vi "Initialize Acquisition.vi"(8 "error in":errorcluster, 11 "DAQmxChannel":T1) -> (0 "error out":errorcluster, 3 "task out":refnum<k21>)   [LabVIEW 2018]
doc: "Konfiguruje kana³ pomiarowy karty DAQ do pomiaru napiêcia."
uses:
  controls/daqtypedef.ctl
  <vilib>/DAQmx/create/channels.llb/DAQmx Create Channel (AI-Voltage-Basic).vi
  <vilib>/DAQmx/configure/timing.llb/DAQmx Timing (Sample Clock).vi
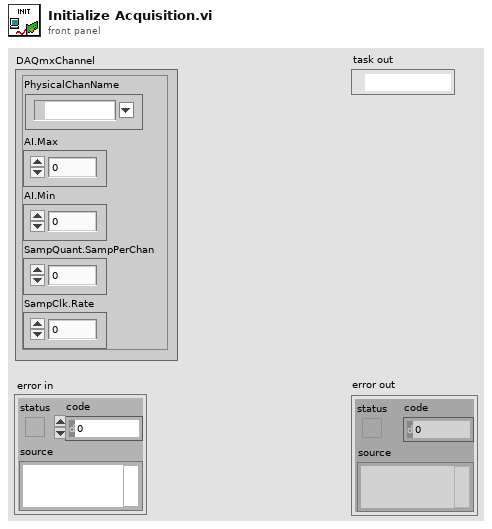
[diagram p1: front panel]
types:
  T1 = typedef "daqtypedef.ctl" = cluster{"PhysicalChanName":tag, "AI.Max":dbl, "AI.Min":dbl, "SampQuant.SampPerChan":dbl, "SampClk.Rate":dbl}
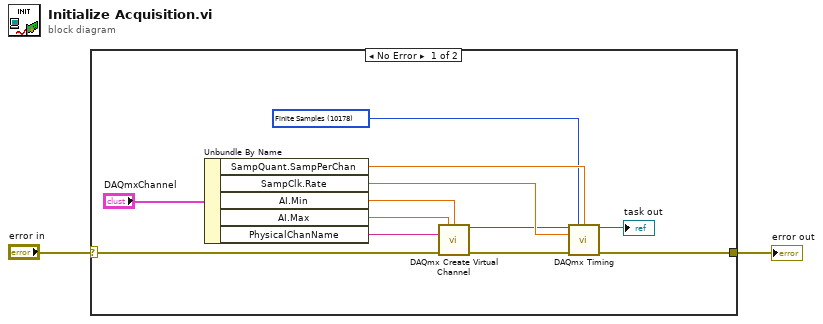
[diagram p0: block diagram]
diagram:
  n1 = case shown="No Error" "error in" {
    selector: "error in" -> [w4 w15]
    tunnel: [w5 w15] -> w2
    frame No Error {
      w8 = 10178 items=["Finite Samples"=10178, "Continuous Samples"=10123, "Hardware Timed Single Point"=12522] ("sample mode")
      n2 = Unbundle By Name("DAQmxChannel") -> ("SampQuant.SampPerChan"=w10:dbl, "SampClk.Rate"=w9:dbl, "AI.Min"=w13:dbl, "AI.Max"=w12:dbl, "PhysicalChanName"=w11:tag)
      n3 = call-poly <vilib>:"DAQmx Create Virtual Channel.vi"("maximum value"=w12, "minimum value"=w13, "physical channels"=w11, "error in"=w4) -> ("task out"=w6:refnum<k21>, "error out"=w7:errorcluster)  [unwired: 10 in]
      n4 = call-poly <vilib>:"DAQmx Timing.vi"("task/channels in"=w6, "sample mode"=w8, "samples per channel"=w10, "rate"=w9, "error in"=w7) -> ("task out"=→"task out":refnum<k21>, "error out"=w5:errorcluster)  [unwired: 9 in]
    }
    frame Error {
    }
  }
  "error out" <- w2
